vi "remote_FGV.vi"(7 "remote_mods":T1, 8 "error in":errorcluster, 10 "data":dbl[][](array[numeric]) format="%0.2f") -> (0 "error out":errorcluster)   [LabVIEW 2018]
uses:
  remote_mods.ctl
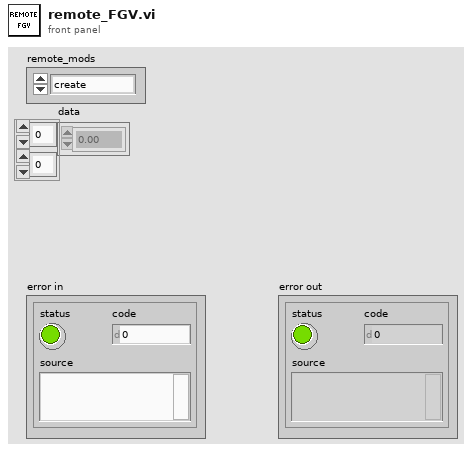
[diagram p1: front panel]
types:
  T1 = typedef "remote_mods.ctl" = enum16{"create", "send", "reconnect", "destroy"}
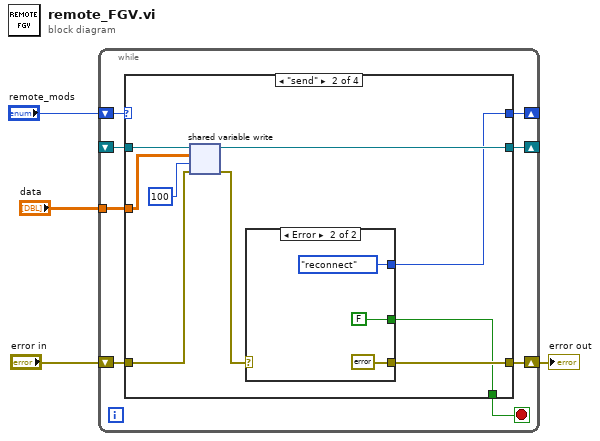
[diagram p0: block diagram]
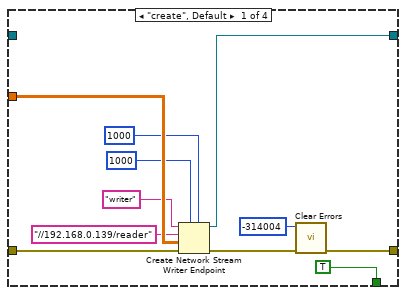
[diagram p2: hidden frame]
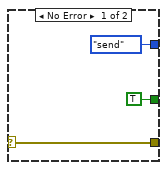
[diagram p3: hidden frame]
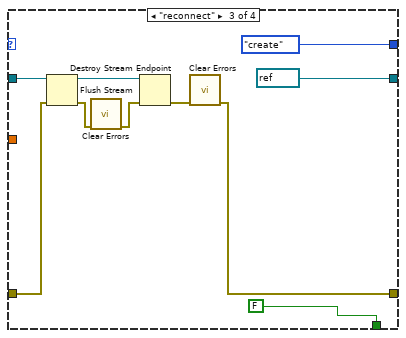
[diagram p4: hidden frame]
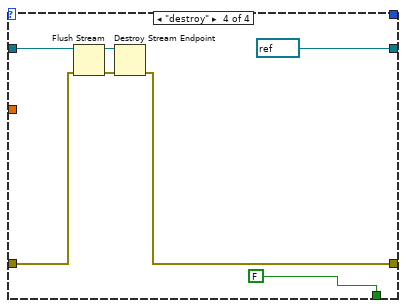
[diagram p5: hidden frame]
diagram:
  n1 = while {
    shift-right: [w5] -> _
    shift-left: "remote_mods" -> [w11]
    shift-right: [w10] -> _
    shift-left: _ -> [w8]
    shift-right: [w9] -> w2
    shift-left: "error in" -> [w12]
    tunnel: "data" -> [w6]
    stop <- w7 stop-if-true
    n2 = case shown="\"send\"" w11 {
      tunnel: w12 -> [w20 w31 w47 w53]
      tunnel: [w19 w30 refnum<k21> refnum ("writer name") refnum<k21> refnum ("writer name")] -> w10
      tunnel: [w13 w26 w41 w52] -> w9
      tunnel: w8 -> [_ w32 w48 w54]
      tunnel: [TRUE w24 FALSE FALSE] -> w7
      tunnel: w6 -> [w23 w29 _ _]
      tunnel: [_ w25 remote_mods."create" ("remote_mods") _] -> w5
      frame "create", Default {
        n3 = Create Network Stream Writer Endpoint(5:1000 ("timeout in ms (-1)"), 7:1000 ("writer buffer size"), 8:w20, 9:w23, 10:"//192.168.0.139/reader" ("reader url"), 11:"writer" ("writer name")) -> (0:w15:errorcluster, 3:w19:refnum<k21>)  [unwired: 1 in]
        n4 = call <vilib>:"Clear Errors.vi"("error in (no error)"=w15, "specific error code to clear (0: all)"=-314004) -> ("error out"=w13:errorcluster)  [unwired: 4 in, 1 out]
      }
      frame "send" {
        n5 = shared-variable-write(w32, w31, w29, 100 ("timeout ms (-1)")) -> (w30:refnum<k21>, w27:errorcluster)  [unwired: 1 out]
        n6 = case shown="Error" w27 {
          selector: w27 -> [w35 _]
          tunnel: [w35 errorcluster {"status"=FALSE, "code"=0, "source"=""} ("error IO")] -> w26
          tunnel: [remote_mods."send" ("remote_mods") remote_mods."reconnect" ("remote_mods")] -> w25
          tunnel: [TRUE FALSE] -> w24
          frame No Error {
          }
          frame Error {
          }
        }
      }
      frame "reconnect" {
        n7 = Flush Stream(8:w47, 11:w48) -> (0:w46:errorcluster, 3:w45:refnum<k21>)  [unwired: 2 in, 1 out]
        n8 = call <vilib>:"Clear Errors.vi"("error in (no error)"=w46) -> ("error out"=w44:errorcluster)  [unwired: 5 in, 1 out]
        n9 = Destroy Stream Endpoint(8:w44, 11:w45) -> (0:w43:errorcluster)
        n10 = call <vilib>:"Clear Errors.vi"("error in (no error)"=w43) -> ("error out"=w41:errorcluster)  [unwired: 5 in, 1 out]
      }
      frame "destroy" {
        n11 = Flush Stream(8:w53, 11:w54) -> (0:w51:errorcluster, 3:w55:refnum<k21>)  [unwired: 2 in, 1 out]
        n12 = Destroy Stream Endpoint(8:w51, 11:w55) -> (0:w52:errorcluster)
      }
    }
  }
  "error out" <- w2
